vi "Do.vi"(8 "error in (no error)":errorcluster, 10 "Actor in":refnum<class "Actor.lvclass">, 11 "Change Panel Msg in":refnum<class "Change Panel Msg.lvclass">) -> (0 "error out":errorcluster, 2 "Actor out":refnum<class "Actor.lvclass">)   [LabVIEW 2023, in "Panel Actor.lvlib" / "Change Panel Msg.lvclass"]
doc: "(<B>Filename</B>: Actor Framework.lvlib:Message.lvclass:Do.vi)\n\nDefines what a message does when it is received by an actor. Generally, a message instructs an actor to invoke one of its methods. By default, this method does nothing. A child class must override it to define behavior. Create a child class by using the Actor Framework Message Maker dialog box."
uses:
  Change Panel Msg.lvclass
  builds/Framework/Actor Framework.lvlibp/1abvi3w/vi.lib/ActorFramework/Actor/Actor.lvclass
  Library/Panel Actor.lvclass
  C:/Users/Public/Documents/Development/builds/Framework/Actor Framework.lvlibp/1abvi3w/vi.lib/ActorFramework/Actor/Actor.lvclass
  Change Panel Msg.lvclass/Change Panel Msg.ctl
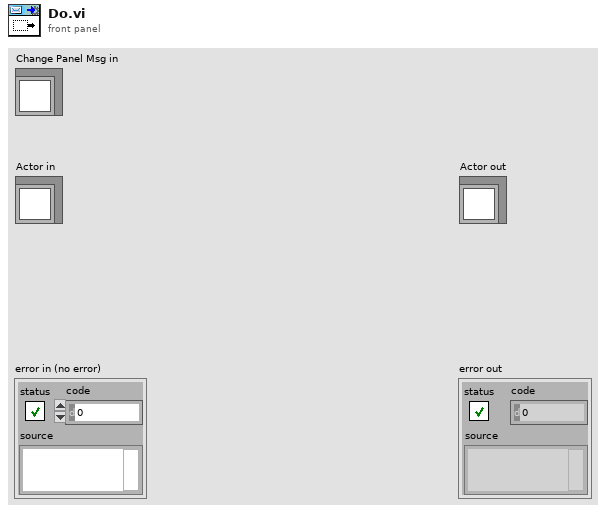
[diagram p1: front panel]
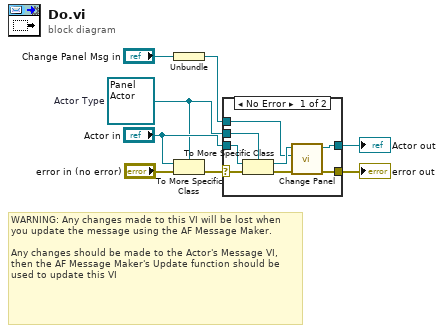
[diagram p0: block diagram]
diagram:
  w3 = refnum<class "Panel Actor.lvclass"> refnum  # Actor Type
  # "WARNING: Any changes made to this VI will be lost when you update the message using the AF Message Maker.\n\nAny changes should be made to the Actor's Message VI, then the AF Message Maker's Update function should be used to update this VI"
  n1 = Unbundle("Change Panel Msg in") -> (w2:refnum<class "Panel.lvclass">)
  n2 = To More Specific Class(target class=w3, reference="Actor in", error in="error in (no error)") -> (error out=w7:errorcluster)  [unwired: 1 out]
  n3 = case shown="No Error" w7 {
    selector: w7 -> [w16 w18]
    tunnel: [w11 w18] -> w6
    tunnel: [w10 w17] -> w5
    tunnel: "Actor in" -> [w15 w17]
    tunnel: w3 -> [w14 _]
    tunnel: w2 -> [w9 _]
    frame No Error {
      n4 = To More Specific Class ("Actor Cast")(target class=w14, reference=w15, error in=w16) -> (specific class reference=w13:refnum<class "Panel Actor.lvclass">, error out=w12:errorcluster)
      n5 = call "Change Panel.vi"("error in (no error)"=w12, "New Panel"=w9, "Panel Actor in"=w13) -> ("error out"=w11:errorcluster, "Panel Actor out"=w10:refnum<class "Panel Actor.lvclass">)  [unwired: 7 in]
    }
    frame Error {
    }
  }
  "error out" <- w6
  "Actor out" <- w5
